vi "Parse and Scale Slip Data.vi"(11 "Slip cluster In":T1) -> (3 "Slip Cluster Out":T1)   [LabVIEW 2020]
uses:
  SlipDataCluster.ctl
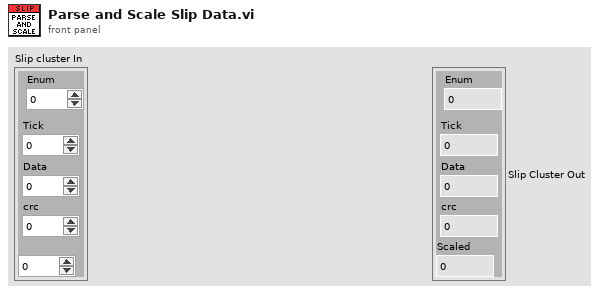
[diagram p1: front panel]
types:
  T1 = typedef "SlipDataCluster.ctl" = cluster{"Enum":u16, "Tick":u32, "Data":u32, "crc":u16, "Scaled":dbl}
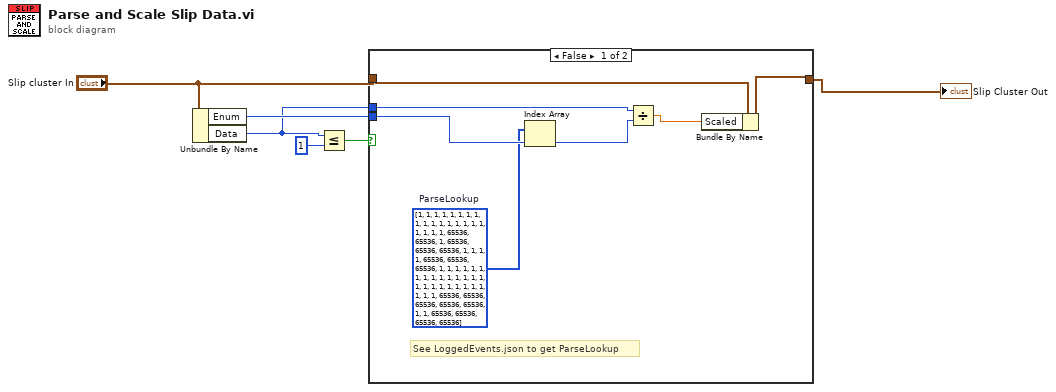
[diagram p0: block diagram]
diagram:
  n1 = Unbundle By Name("Slip cluster In") -> ("Enum"=w2:u16, "Data"=w1:u32)
  n2 = Less Or Equal?(x=w1, y=u32 1) -> (x <= y?=w3:bool)
  n3 = case shown="False" w3 {
    tunnel: [w13 w14] -> w6
    tunnel: "Slip cluster In" -> [w12 w14]
    tunnel: w2 -> [w11 _]
    tunnel: w1 -> [w8 _]
    frame False {
      w10 = u32[] [1, 1, 1, 1, 1, 1, 1, 1, 1, 1, 1, 1, 1, 1, 1, 1, 1, 1, 1, 1, 1, 65536, 65536, 1, 65536, 65536, 65536, 1, 1, 1, 1, 65536, 65536, 65536, 1, 1, 1, 1, 1, 1, 1, 1, 1, 1, 1, 1, 1, 1, 1, 1, 1, 1, 1, 1, 1, 1, 1, 1, 1, 1, 1, 65536, 65536, 65536, 65536, 65536, 1, 1, 65536, 65536, 65536, 65536]  # ParseLookup
      # "See LoggedEvents.json to get ParseLookup"
      n4 = Index Array(array=w10, index=w11) -> (element=w9:u32)
      n5 = Divide(x=w8, y=w9) -> (x/y=w7:dbl)
      n6 = Bundle By Name(cluster=w12, "Scaled"=w7) -> (w13:T1)
    }
    frame True {
    }
  }
  "Slip Cluster Out" <- w6
